vi "VFP Alarming Validate Unique Name.vi"(10 "Names Array":string[](array[string]), 11 "Enabled Array":bool[](array[boolean])) -> (2 "Confliction Name":string, 3 "Validate?":bool)   [LabVIEW 2016]
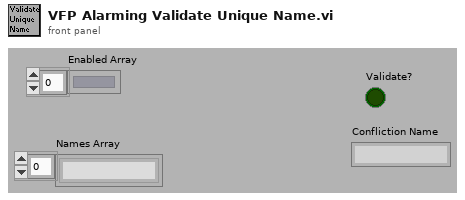
[diagram p1: front panel]
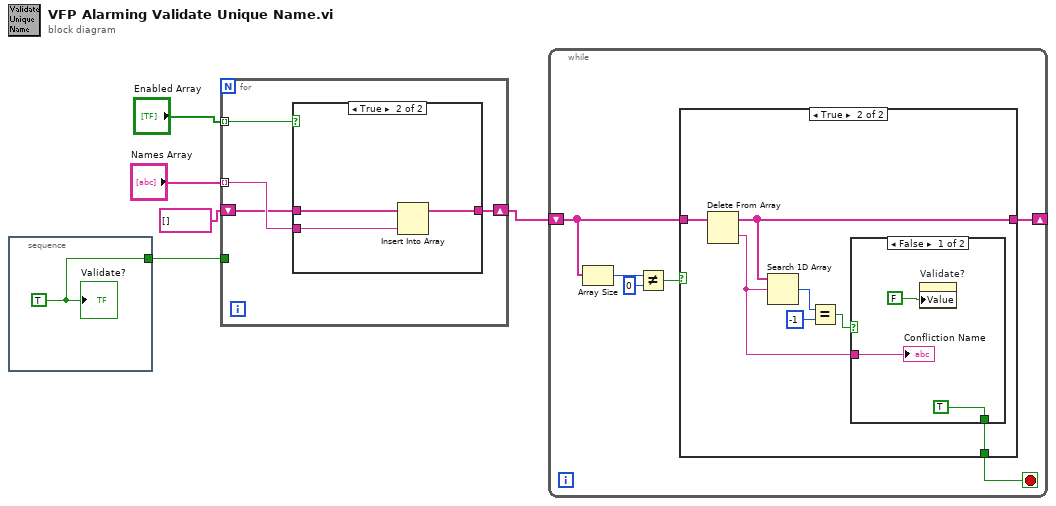
[diagram p0: block diagram]
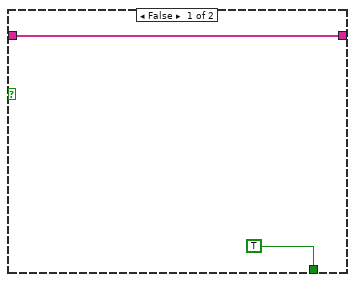
[diagram p2: hidden frame]
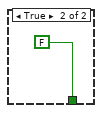
[diagram p3: hidden frame]
diagram:
  n1 = stacked-sequence {
    tunnel: [w6] -> w2
    frame #0 {
      w6 = TRUE ("Boolean")
      "Validate?" <- w6
    }
  }
  n2 = for {
    tunnel: "Enabled Array" -> [w10] mode=indexing
    tunnel: "Names Array" -> [w9] mode=indexing
    shift-right: [w8] -> w1
    shift-left: string[] [] -> [w7]
    tunnel: w2 -> [_]
    n3 = case shown="True" w10 {
      tunnel: w9 -> [_ w14]
      tunnel: [w11 w13] -> w8
      tunnel: w7 -> [w11 w12]
      frame False {
      }
      frame True {
        n4 = Insert Into Array(array=w12, new element=w14) -> (w13:string[])  [unwired: 1 in]
      }
    }
  }
  n5 = while {
    shift-right: [w15] -> _
    shift-left: w1 -> [w16]
    stop <- w17 stop-if-true
    n6 = Array Size(array=w16) -> (size(s)=w20:i32)
    n7 = Not Equal?(x=w20, y=0) -> (x != y?=w18:bool)
    n8 = case shown="True" w18 {
      tunnel: [TRUE w24] -> w17
      tunnel: w16 -> [w21 w29]
      tunnel: [w21 w28] -> w15
      frame False {
      }
      frame True {
        n9 = Delete From Array(array=w29) -> (deleted portion=w23:string, array with subset deleted=w28:string[])  [unwired: 2 in]
        n10 = Search 1D Array(1D array=w28, element=w23) -> (index of element=w27:i32)  [unwired: 1 in]
        n11 = Equal?(x=w27, y=-1) -> (x = y?=w25:bool)
        n12 = case shown="False" w25 {
          tunnel: [TRUE FALSE] -> w24
          tunnel: w23 -> [w30 _]
          frame False {
            n13 = property on="Validate?" class="Bool (strict)"("Value"=FALSE ("Validate?")) -> ()  [unwired: 2 in, 2 out]
            "Confliction Name" <- w30
          }
          frame True {
          }
        }
      }
    }
  }
